vi "Temperature serial v7.vi"(0 "Command String":string, 5 "Time Out (S)":dbl=0.5, 7 "CALIB":dbl) -> (4 "T1":dbl, 6 "T2":dbl, 8 "T3":dbl, 10 "T4":dbl, 13 "error":bool, 14 "output cluster":cluster{dbl, dbl, dbl, dbl, i32, "error #":dbl}, 15 "Unit ID":dbl)   [LabVIEW 2017]
uses:
  program files/Global 1.vi
panel:
  out "Retry":i32
  out "error out":errorcluster
  out "COM port":refnum<visa-resource-name>="COM6"
  out "error #":dbl
  out "End T":dbl
  out "Start T":dbl
  out "read time":u64
  in  "Array - String":string[](array[string])
  out "end of data (#)":bool
  out "data bytes read":dbl
  out "data string":string
  out "read buffer":string
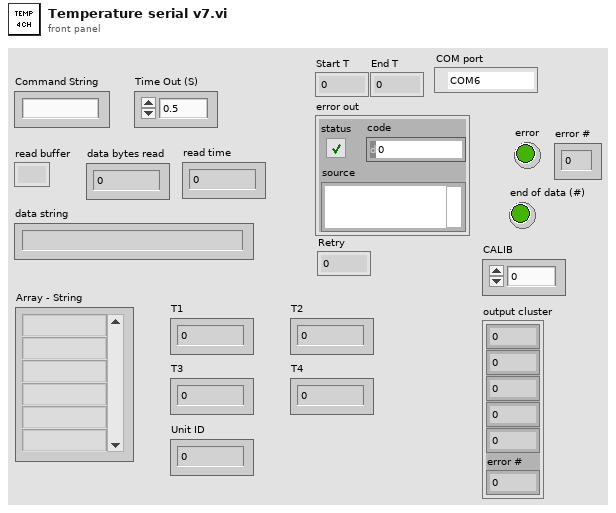
[diagram p1: front panel]
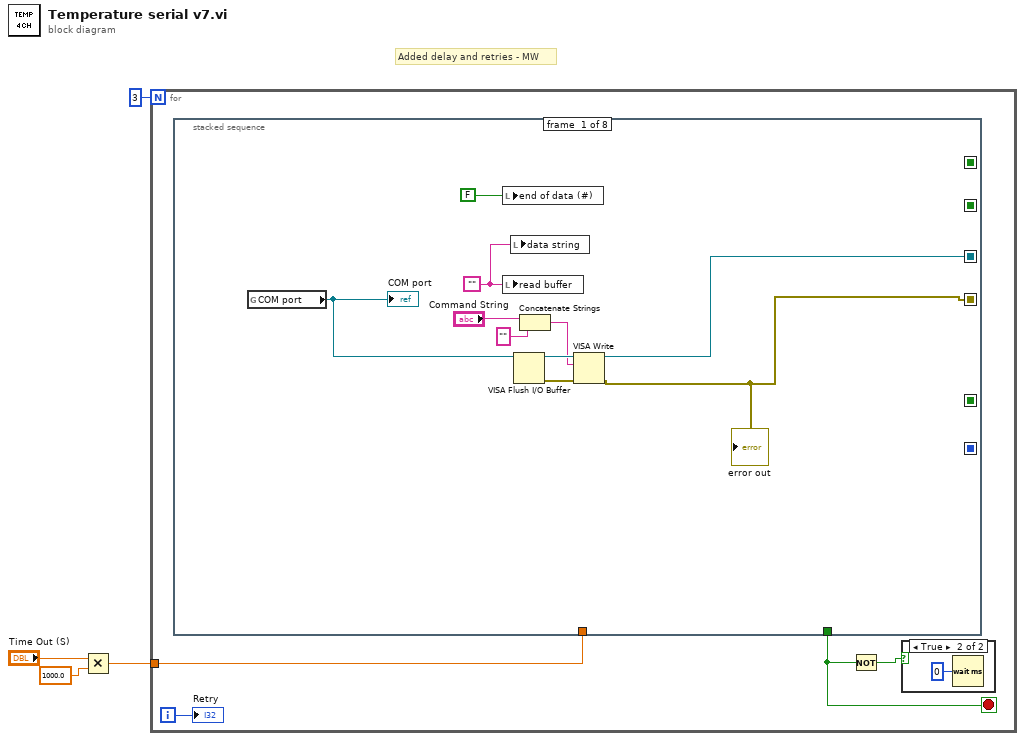
[diagram p0: block diagram]
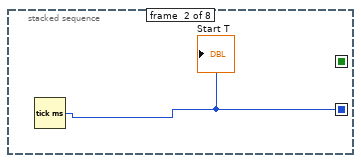
[diagram p3: hidden frame]
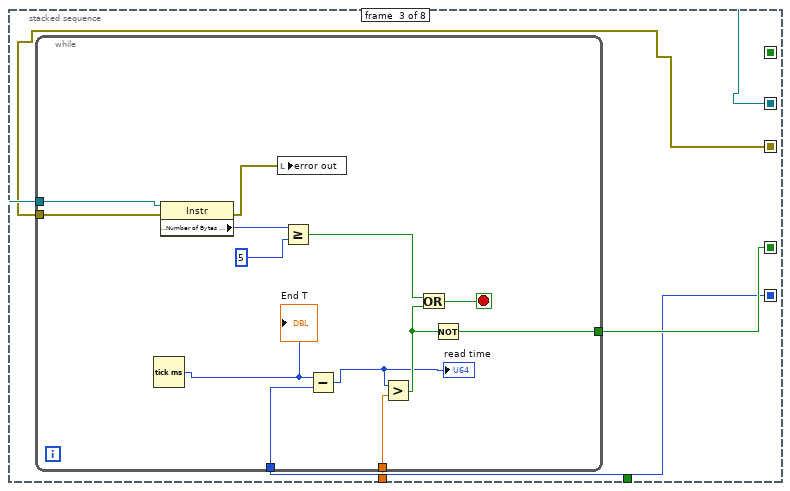
[diagram p4: hidden frame]
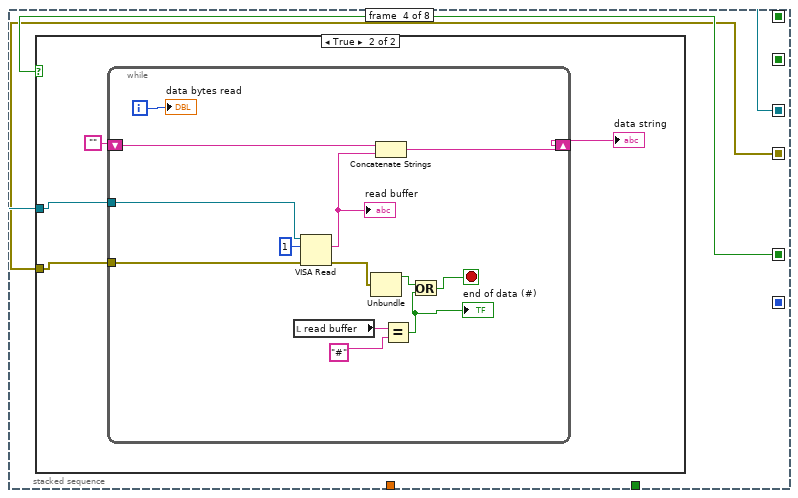
[diagram p5: hidden frame]
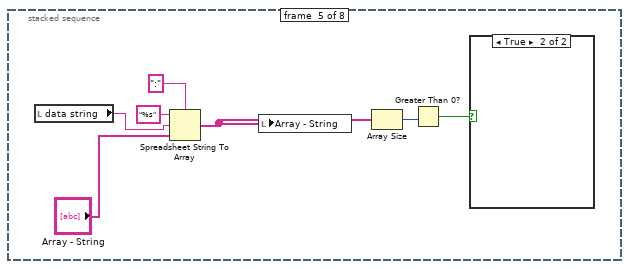
[diagram p7: hidden frame]
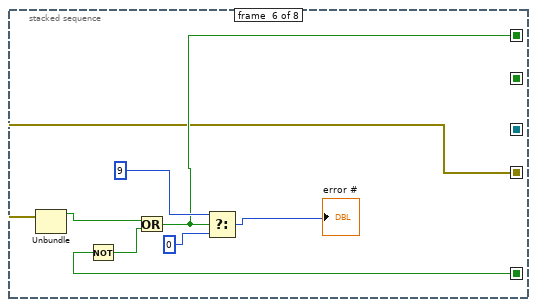
[diagram p9: hidden frame]
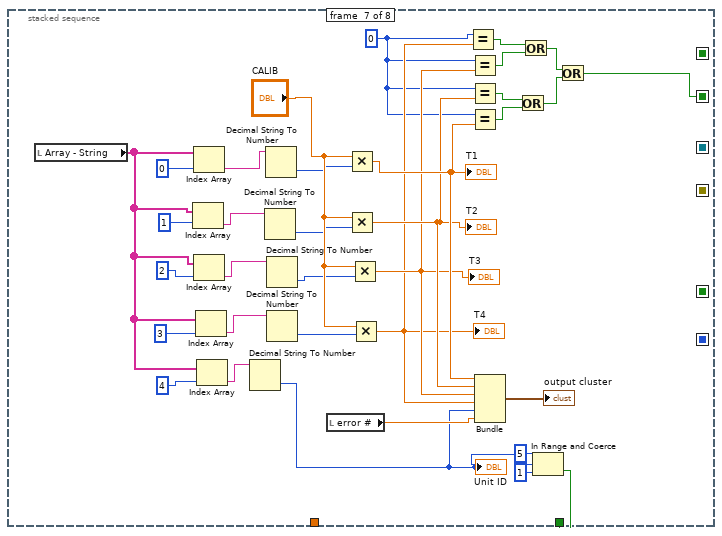
[diagram p10: hidden frame]
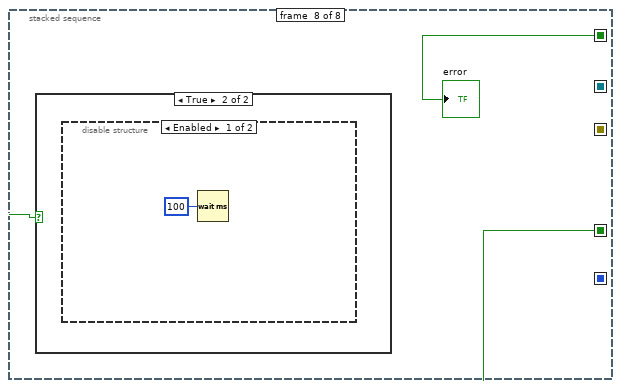
[diagram p11: hidden frame]
diagram:
  # "Added delay and retries - MW"
  n1 = Multiply(x="Time Out (S)", y=1000.0) -> (x*y=w1:dbl)
  n2 = for {
    N: 3 -> [_]
    tunnel: w1 -> [w5]
    i -> [w8]
    stop <- w7 stop-if-true
    n3 = stacked-sequence {
      seq-local: [_ _ w25 _ _ _ _ _] -> [_ _ _ w41 _ w72 _ w108]
      seq-local: [_ w20 _ _ _ _ _ _] -> [_ _ w24 _ _ _ _ _]
      seq-local: [_ _ _ _ _ w67 _ _] -> [_ _ _ _ _ _ _ _]
      seq-local: [_ _ _ _ _ _ w78 _] -> [_ _ _ _ _ _ _ w109]
      seq-local: [w14 _ _ _ _ _ _ _] -> [_ _ w23 w40 _ _ _ _]
      seq-local: [w13 _ _ _ _ _ _ _] -> [_ _ w22 w39 _ w66 _ _]
      tunnel: [_ _ _ _ _ _ w74 _] -> w7
      tunnel: w5 -> [_ _ w21 _ _ _ _ _]
      frame #0 {
        w19 = ""
        n4 = global read "Global 1.vi" "COM port"() -> (w15:refnum<visa-resource-name>)
        "COM port" <- w15
        n5 = local write "end of data (#)"(FALSE) -> ()
        n6 = local write "read buffer"(w19) -> ()
        n7 = local write "data string"(w19) -> ()
        n8 = VISA Flush I/O Buffer(VISA resource name=w15) -> (VISA resource name out=w17:refnum<visa-resource-name>, error out=w16:errorcluster)  [unwired: 2 in]
        n9 = Concatenate Strings("Command String", "" ("string")) -> (w10:string)
        n10 = VISA Write(VISA resource name=w17, write buffer=w10, error in (no error)=w16) -> (VISA resource name out=w14:refnum<visa-resource-name>, error out=w13:errorcluster)  [unwired: 1 out]
        "error out" <- w13
      }
      frame #1 {
        n11 = Tick Count (ms)() -> (millisecond timer value=w20:u32)
        "Start T" <- w20
      }
      frame #2 {
        n12 = while {
          tunnel: w23 -> [w38]
          tunnel: w22 -> [w37]
          tunnel: [w30] -> w25
          tunnel: w24 -> [w33]
          tunnel: w21 -> [w26]
          stop <- w32 stop-if-true
          n13 = Tick Count (ms)() -> (millisecond timer value=w28:u32)
          "End T" <- w28
          n14 = property class="Instr"(reference=w38, error in=w37) -> (error out=w34:errorcluster, "Serial Settings:Number of Bytes at Serial Port"=w36:u32)  [unwired: 1 out]
          n15 = local write "error out"(w34) -> ()
          n16 = Greater Or Equal?(x=w36, y=5) -> (x >= y?=w29:bool)
          n17 = Subtract(x=w28, y=w33) -> (x-y=w27:u32)
          "read time" <- w27
          n18 = Greater?(x=w27, y=w26) -> (0:w31:bool)
          n19 = Or(x=w29, y=w31) -> (x .or. y?=w32:bool)
          n20 = Not(x=w31) -> (.not. x?=w30:bool)
        }
      }
      frame #3 {
        n21 = case shown="True" w41 {
          tunnel: w40 -> [_ w45]
          tunnel: w39 -> [_ w44]
          frame False {
          }
          frame True {
            n22 = while {
              tunnel: w45 -> [w53]
              tunnel: w44 -> [w52]
              shift-right: [w51] -> w43
              shift-left: "" -> [w50]
              i -> [w54]
              stop <- w46 stop-if-true
              n23 = local read "read buffer"() -> (w57:string)
              n24 = VISA Read(VISA resource name=w53, byte count=u32 1, error in (no error)=w52) -> (read buffer=w55:string, error out=w49:errorcluster)  [unwired: 2 out]
              "read buffer" <- w55
              n25 = Unbundle(w49) -> ("status"=w48:bool)  [unwired: 2 out]
              n26 = Concatenate Strings(w50, w55) -> (w51:string)
              n27 = Equal?(x=w57, y="#") -> (x = y?=w47:bool)
              "end of data (#)" <- w47
              n28 = Or(x=w48, y=w47) -> (x .or. y?=w46:bool)
              "data bytes read" <- w54
            }
            "data string" <- w43
          }
        }
      }
      frame #4 {
        n29 = local read "data string"() -> (w63:string)
        n30 = Spreadsheet String To Array(delimiter (Tab)=":", format string="%s", spreadsheet string=w63, array type (2D Dbl)="Array - String") -> (array=w61:string[])
        n31 = local write "Array - String"(w61) -> ()
        n32 = Array Size(array=w61) -> (size(s)=w60:i32)
        n33 = Greater Than 0?(x=w60) -> (x > 0?=w59:bool)
        n34 = case shown="True" w59 {
          frame False {
          }
          frame True {
          }
        }
      }
      frame #5 {
        n35 = Unbundle(w66) -> ("status"=w73:bool)  [unwired: 2 out]
        n36 = Not(x=w72) -> (.not. x?=w71:bool)
        n37 = Or(x=w73, y=w71) -> (x .or. y?=w67:bool)
        n38 = Select(t=9, s=w67, f=0) -> (s? t:f=→"error #":i32)
      }
      frame #6 {
        w85 = 0
        n39 = local read "Array - String"() -> (w99:string[])
        n40 = Index Array(array=w99, index=1) -> (element=w102:string)
        n41 = Index Array(array=w99, index=0) -> (element=w106:string)
        n42 = Index Array(array=w99, index=2) -> (element=w101:string)
        n43 = Index Array(array=w99, index=3) -> (element=w100:string)
        n44 = Index Array(array=w99, index=4) -> (element=w97:string)
        n45 = Decimal String To Number(string=w97) -> (number=w77:i32)  [unwired: 2 in, 1 out]
        "Unit ID" <- w77
        n46 = Decimal String To Number(string=w102) -> (number=w94:i32)  [unwired: 2 in, 1 out]
        n47 = Decimal String To Number(string=w106) -> (number=w95:i32)  [unwired: 2 in, 1 out]
        n48 = Decimal String To Number(string=w101) -> (number=w93:i32)  [unwired: 2 in, 1 out]
        n49 = Decimal String To Number(string=w100) -> (number=w92:i32)  [unwired: 2 in, 1 out]
        n50 = local read "error #"() -> (w91:dbl)
        n51 = Multiply(x="CALIB", y=w95) -> (x*y=w89:dbl)
        "T1" <- w89
        n52 = Multiply(x="CALIB", y=w94) -> (x*y=w88:dbl)
        "T2" <- w88
        n53 = Multiply(x="CALIB", y=w93) -> (x*y=w87:dbl)
        "T3" <- w87
        n54 = Multiply(x="CALIB", y=w92) -> (x*y=w86:dbl)
        "T4" <- w86
        n55 = Equal?(x=w85, y=w86) -> (x = y?=w81:bool)
        n56 = Equal?(x=w85, y=w87) -> (x = y?=w82:bool)
        n57 = Equal?(x=w85, y=w88) -> (x = y?=w84:bool)
        n58 = Equal?(x=w85, y=w89) -> (x = y?=w83:bool)
        n59 = Bundle(w89, w88, w87, w86, w77, "error #"=w91) -> (→"output cluster":cluster{dbl, dbl, dbl, dbl, i32, "error #":dbl})  [unwired: 1 in]
        n60 = Or(x=w84, y=w83) -> (x .or. y?=w79:bool)
        n61 = Or(x=w81, y=w82) -> (x .or. y?=w80:bool)
        n62 = In Range and Coerce(upper limit=5, x=w77, lower limit=1) -> (In Range?=w74:bool)  [unwired: 1 out]
        n63 = Or(x=w80, y=w79) -> (x .or. y?=w78:bool)
      }
      frame #7 {
        n64 = case shown="True" w108 {
          frame False {
          }
          frame True {
            n65 = disable-structure shown="Enabled" {
              frame Enabled {
                n66 = Wait (ms)(milliseconds to wait=u32 100) -> ()  [unwired: 1 out]
              }
              frame Disabled {
              }
            }
          }
        }
        "error" <- w109
      }
    }
    n67 = Not(x=w7) -> (.not. x?=w6:bool)
    n68 = case shown="True" w6 {
      frame False {
      }
      frame True {
        n69 = Wait (ms)(milliseconds to wait=u32 0) -> ()  [unwired: 1 out]
      }
    }
    "Retry" <- w8
  }
